vi "tsdb_get_lin_db_id.vi"(8 "error in (no error)":errorcluster caption="错误输入（无错误）", 11 "AIndex":i32) -> (0 "error out":errorcluster caption="错误输出", 2 "AId":u32, 3 "return":i32)   [LabVIEW 2014]
doc: "Function Introduction ：\nGet LIN database ID\nCall location ：\ninput parameter ：\nAIdex: Database Index\nAId: Returned database ID\nReturn value ：\n==0: Execution successful\nOther values: Query error code"
panel:
  out "path out":path
  in  "path in":path
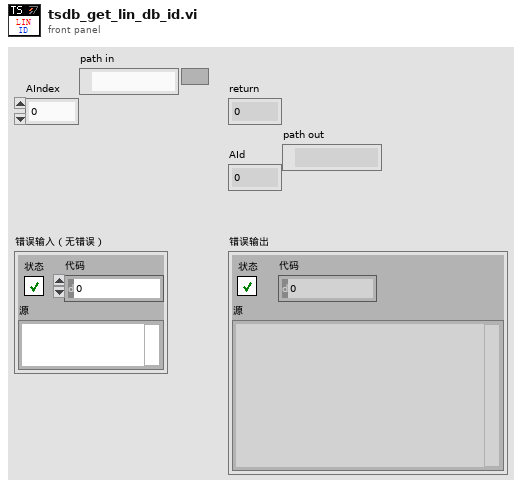
[diagram p1: front panel]
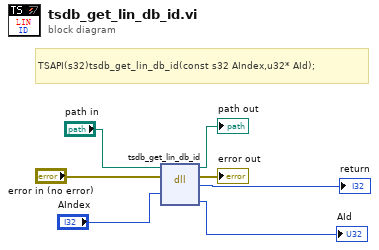
[diagram p0: block diagram]
diagram:
  # "TSAPI(s32)tsdb_get_lin_db_id(const s32 AIndex,u32* AId);"
  n1 = dll-call lib="D:/Program Files (x86)/TOSUN/TSMaster/bin64/TSMaster.dll" fn="tsdb_get_lin_db_id"(path in="path in", error in="error in (no error)", "AIndex"="AIndex") -> (path out=→"path out":path, error out=→"error out":errorcluster, "return type"=→"return":i32, "AId"=→"AId":u32)  [unwired: 3 in]
